vi "Ballard 429 - Parse Message.vi"(8 "Error (in)":errorcluster, 9 "Data (in)":dbl[](array[numeric]), 10 "Record []":T13[](array[typedef]) {"type" format="%04x"; "timestamp" format="%08x"; "msgact" format="%04x"; "data" format="%08x"; "timestamph" format="%08x"}, 11 "Channel Data []":T1[](array[typedef])=[{"Labels Settings"=[{"Name"="", "xmlName"="", "Label"=0, "transferPeriod"=0, "Driver Data"={"Lbl Tx Hdl"=0, "Decimation"=0, "IterationOffset"=0, "transfer handle"=0, "RX Word"=0, "TXChange"=FALSE, "RX timestamp"=0.0}, "SDI_Enabled"=FALSE, "SDI"=0, "Words"=[{"Block Data Refs"=[], "Values Array"=[], "Length"=0, "FIFO Index"=0, "Param Setting"={"Start Bit"=[1], "Num Bits"=[], "Signed?"=[], "ScaleFac"=[], "ScaleOffset"=[], "Channel FIFO Buffer Index"=[]}}], "bufferSize"=0, "RxWordIdx"=0, "TxWordIdx"=0, "TransferType"=enum."ScheduledLabel", "has timestamp?"=FALSE, "LBL Disable Index"=0, "Message Handle"=0, "Initialized?"=FALSE}], "channel handle"=0, "channel #"=0, "Label Map"=[], "Label Buffer"=[], "rdBufHandle"=0}] {"Labels Settings"."Label" format="%.0o"}) -> (0 "Error (out)":errorcluster, 1 "Doubles []":dbl[](array[numeric]))   [LabVIEW 2017, in "Ballard Arinc-429 Engine.lvlib"]
uses:
  Ballard Arinc-429 Engine.lvlib
  <instrlib>/BTICardLib/Public/Controls/429 Record.ctl
  RT Controls/RT HW Channel.ctl
  RT Controls/RT Label Settings.ctl
  Shared/Controls and Global/Label.ctl
  Shared/Controls and Global/transferPeriod.ctl
  RT Controls/Driver Data.ctl
  RT Controls/RT Word Settings.ctl
  <vilib>/NI Veristand/Custom Device API/Block Data Reference.ctl
  <vilib>/NI Veristand/Custom Device API/Data Reference.ctl
  RT Controls/RT Param Setting.ctl
  Shared/Controls and Global/Start Bit.ctl
  Shared/Controls and Global/Number of Bits.ctl
  Shared/Controls and Global/TransferType.ctl
  <instrlib>/BTI429Lib/BTI429LV.lvlib
  Shared/Ballard Arinc-429 Shared.lvlib
  <instrlib>/BTI429Lib/Private/Utility/Get Fld SDI.vi
  <instrlib>/BTICardLib/BTICardLV.lvlib
  <vilib>/NI Veristand/Custom Device API/Custom Device API.lvlib
panel:
  out "Waveform Chart":i32(graph)
  out "source/destination identifiers (SDI) out":u8 format="%02b"
  out "Label #":i32
  out "Physical Channel #":i32
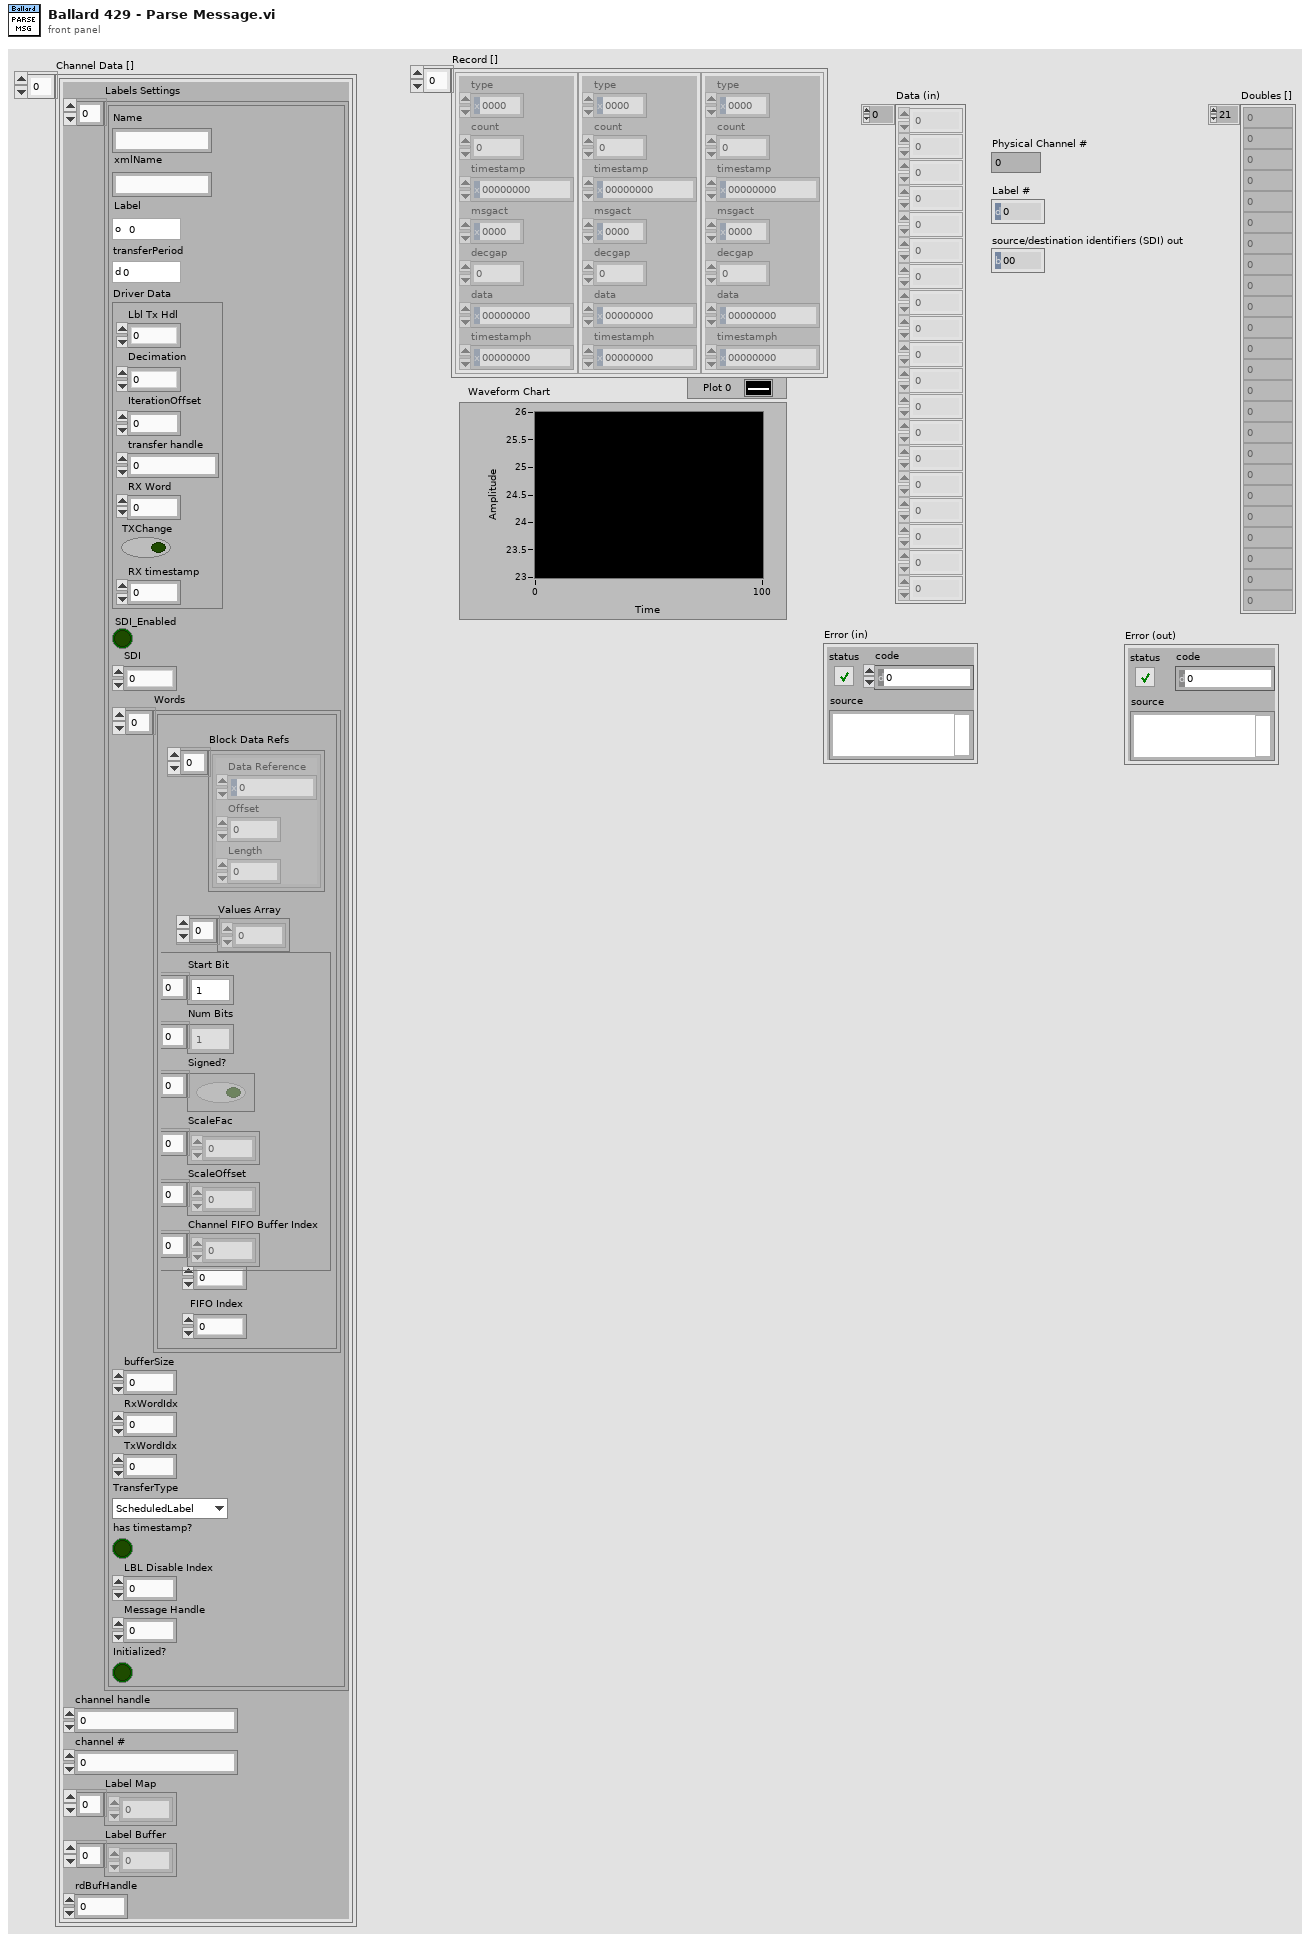
[diagram p1: front panel]
types:
  T1 = typedef "Ballard Arinc-429 Engine.lvlib/RT HW Channel.ctl" = cluster{"Labels Settings":T2[], "channel handle":u32, "channel #":u16, "Label Map":i32[], "Label Buffer":u32[], "rdBufHandle":u32}
  T2 = typedef "Ballard Arinc-429 Engine.lvlib/RT Label Settings.ctl" = cluster{"Name":string, "xmlName":string, "Label":T3, "transferPeriod":T4, "Driver Data":T5, "SDI_Enabled":bool, "SDI":u8, "Words":T6[], "bufferSize":u32, "RxWordIdx":i32, "TxWordIdx":i32, "TransferType":T12, "has timestamp?":bool, "LBL Disable Index":i32, "Message Handle":u64, "Initialized?":bool}
  T3 = typedef "Ballard Arinc-429 Shared.lvlib/Label.ctl" = u8
  T4 = typedef "Ballard Arinc-429 Shared.lvlib/transferPeriod.ctl" = u32
  T5 = typedef "Ballard Arinc-429 Engine.lvlib/Driver Data.ctl" = cluster{"Lbl Tx Hdl":u32, "Decimation":i32, "IterationOffset":i32, "transfer handle":u32, "RX Word":u32, "TXChange":bool, "RX timestamp":dbl}
  T6 = typedef "Ballard Arinc-429 Engine.lvlib/RT Word Settings.ctl" = cluster{"Block Data Refs":T7[], "Values Array":dbl[], "Length":i32, "FIFO Index":i32, "Param Setting":T9}
  T7 = typedef "Custom Device API.lvlib/Block Data Reference.ctl" = cluster{"Data Reference":T8, "Offset":u64, "Length":u64}
  T8 = typedef "Custom Device API.lvlib/Data Reference.ctl" = i32
  T9 = typedef "Ballard Arinc-429 Engine.lvlib/RT Param Setting.ctl" = cluster{"Start Bit":T10[], "Num Bits":T11[], "Signed?":bool[], "ScaleFac":dbl[], "ScaleOffset":dbl[], "Channel FIFO Buffer Index":i32[]}
  T10 = typedef "Ballard Arinc-429 Shared.lvlib/Start Bit.ctl" = i32
  T11 = typedef "Ballard Arinc-429 Shared.lvlib/Number of Bits.ctl" = i32
  T12 = typedef "Ballard Arinc-429 Shared.lvlib/TransferType.ctl" = enum16{"ScheduledLabel", "Acyclic", "Block", "Strobe"}
  T13 = typedef "BTICardLV.lvlib/429 Record.ctl" = cluster{"type":u16, "count":u16, "timestamp":u32, "msgact":u16, "decgap":u16, "data":u32, "timestamph":u32}
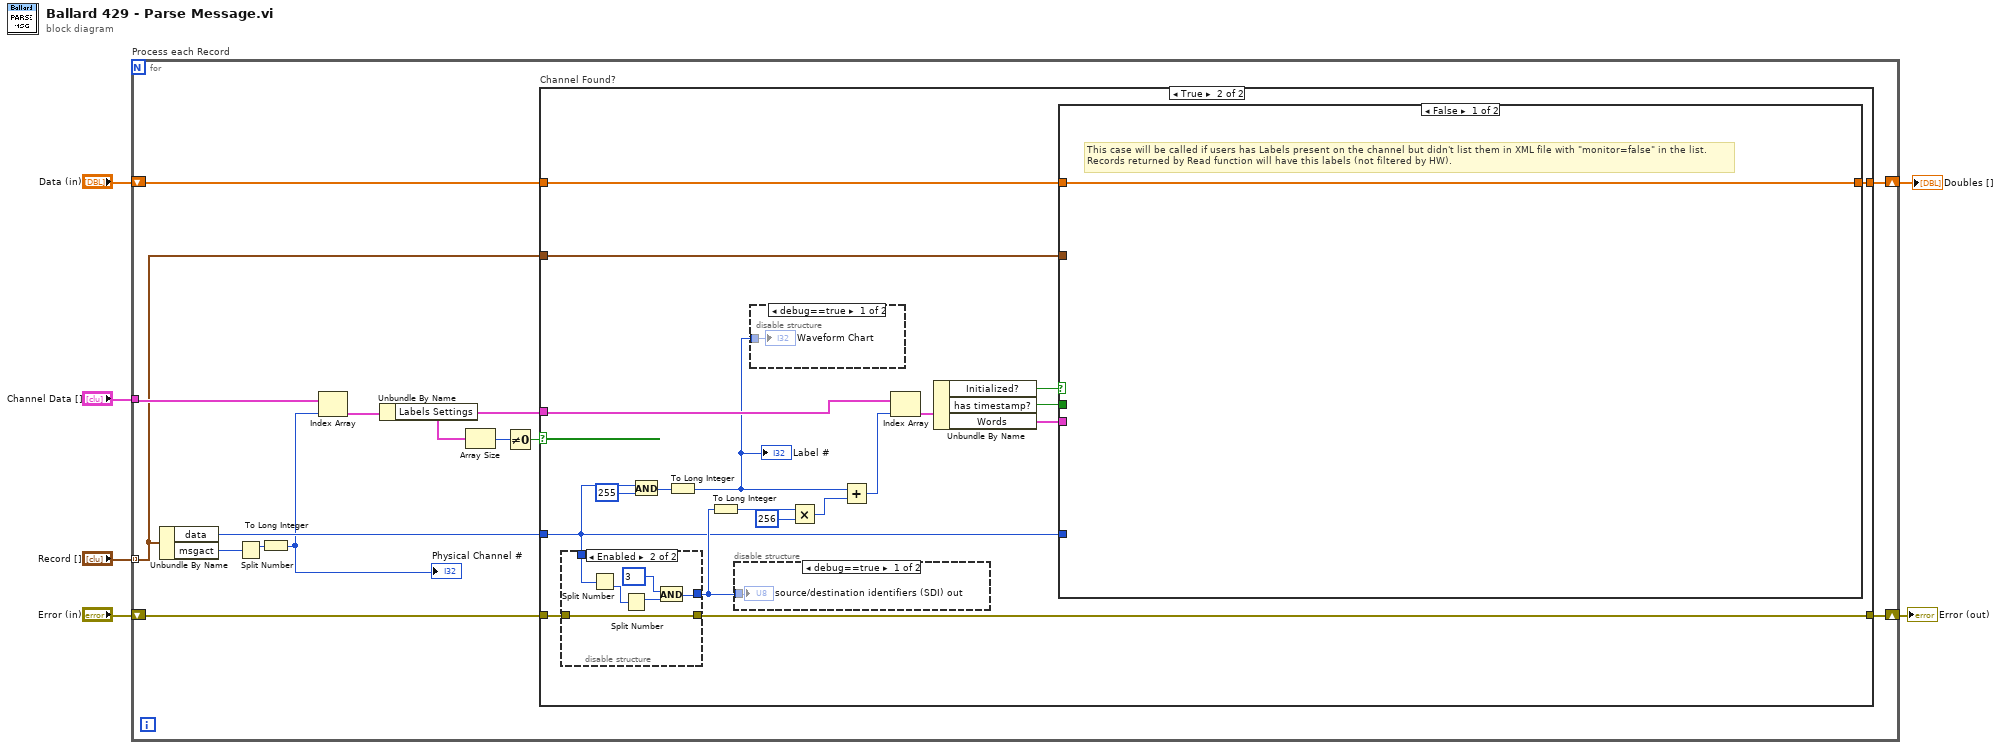
[diagram p0: block diagram]
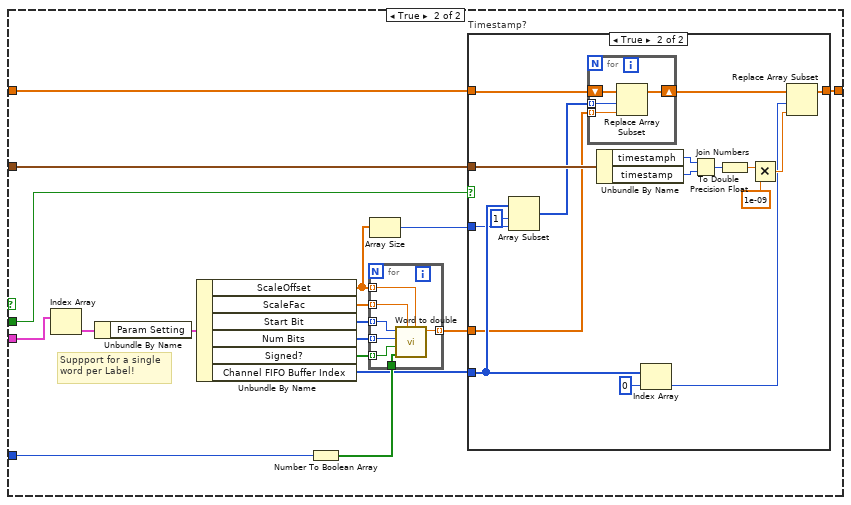
[diagram p3: hidden frame]
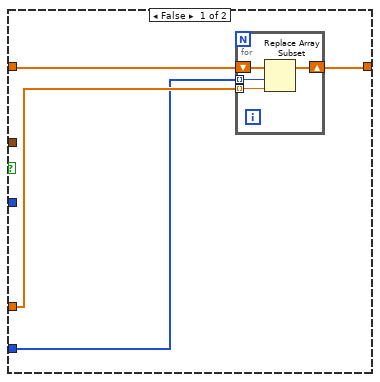
[diagram p4: hidden frame]
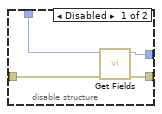
[diagram p7: hidden frame]
diagram:
  n1 = for "Process each Record" {
    tunnel: "Record []" -> [w14] mode=indexing
    shift-right: [w19] -> w3
    shift-left: "Error (in)" -> [w20]
    tunnel: "Channel Data []" -> [w16]
    shift-right: [w7] -> w1
    shift-left: "Data (in)" -> [w11]
    n2 = Unbundle By Name(w14) -> ("data"=w17:u32, "msgact"=w13:u16)
    n3 = Split Number(x=w13) -> (hi(x)=w9:u8)  [unwired: 1 out]
    n4 = To Long Integer(number=w9) -> (32bit integer=w12:i32)
    "Physical Channel #" <- w12
    n5 = Index Array(array=w16, index=w12) -> (element=w15:T1)
    n6 = Unbundle By Name(w15) -> ("Labels Settings"=w8:T2[])
    n7 = Array Size(array=w8) -> (size(s)=w10:i32)
    n8 = Not Equal To 0?(x=w10) -> (x != 0?=w18:bool)
    n9 = case "Channel Found?" shown="True" w18 {
      tunnel: w20 -> [w22 w36]
      tunnel: [w22 w41] -> w19
      tunnel: w17 -> [_ w25]
      tunnel: w14 -> [_ w39]
      tunnel: w11 -> [w21 w27]
      tunnel: w8 -> [_ w33]
      tunnel: [w21 w26] -> w7
      frame False {
      }
      frame True {
        n10 = disable-structure shown="Enabled" {
          disable-tunnel: w25 -> [w101 w106]
          disable-tunnel: w36 -> [w100 w107]
          disable-tunnel: [w99 w107] -> w41
          disable-tunnel: [w98 w104] -> w35
          frame Disabled {
            n11 = call-poly <instrlib>:"Get Fields.vi"("error in (no error)"=w100, "message"=w101) -> ("error out"=w99:errorcluster, "source/destination identifiers (SDI) out"=w98:u16)  [unwired: 8 in]
          }
          frame Enabled {
            n12 = Split Number(x=w106) -> (lo(x)=w105:u16)  [unwired: 1 out]
            n13 = Split Number(x=w105) -> (hi(x)=w103:u8)  [unwired: 1 out]
            n14 = And(x=u8 3, y=w103) -> (x .and. y?=w104:u8)
          }
        }
        n15 = And(x=w25, y=u32 255) -> (x .and. y?=w37:u32)
        n16 = To Long Integer(number=w37) -> (32bit integer=w24:i32)
        "Label #" <- w24
        n17 = To Long Integer(number=w35) -> (32bit integer=w34:i32)
        n18 = disable-structure shown="debug==true" {
          disable-tunnel: w35 -> [w96 _]
          frame condition #0 {
            "source/destination identifiers (SDI) out" <- w96
          }
          frame condition #1 (active) {
          }
        }
        n19 = disable-structure shown="debug==true" {
          disable-tunnel: w24 -> [w97 _]
          frame condition #0 {
            "Waveform Chart" <- w97
          }
          frame condition #1 (active) {
          }
        }
        n20 = Multiply(x=w34, y=256) -> (x*y=w32:i32)
        n21 = Add(x=w24, y=w32) -> (x+y=w31:i32)
        n22 = Index Array(array=w33, index=w31) -> (element=w29:T2)
        n23 = Unbundle By Name(w29) -> ("Initialized?"=w23:bool, "has timestamp?"=w38:bool, "Words"=w40:T6[])
        n24 = case shown="False" w23 {
          tunnel: w40 -> [_ w59]
          tunnel: w39 -> [_ w58]
          tunnel: w38 -> [_ w57]
          tunnel: w27 -> [w42 w49]
          tunnel: [w42 w48] -> w26
          tunnel: w25 -> [_ w47]
          frame False {
            # "This case will be called if users has Labels present on the channel but didn't list them in XML file with \"monitor=false\" in the list.\nRecords returned by Read function will have this labels (not filtered by HW)."
          }
          frame True {
            # "Suppport for a single\nword per Label!"
            n25 = Index Array(array=w59) -> (element=w56:T6)  [unwired: 1 in]
            n26 = Unbundle By Name(w56) -> ("Param Setting"=w55:T9)
            n27 = Unbundle By Name(w55) -> ("ScaleOffset"=w44:dbl[], "ScaleFac"=w54:dbl[], "Start Bit"=w53:T10[], "Num Bits"=w52:T11[], "Signed?"=w51:bool[], "Channel FIFO Buffer Index"=w45:i32[])
            n28 = Number To Boolean Array(number=w47) -> (Boolean array=w46:bool[])
            n29 = for {
              tunnel: [w95] -> w50 mode=indexing
              tunnel: w44 -> [w94] mode=indexing
              tunnel: w54 -> [w93] mode=indexing
              tunnel: w53 -> [w92] mode=indexing
              tunnel: w52 -> [w91] mode=indexing
              tunnel: w51 -> [w90] mode=indexing
              tunnel: w46 -> [w89]
              n30 = call "Word to double.vi"("ScaleOffset (0)"=w94, "ScaleFac (1)"=w93, "Word"=w89, "Signed? (F)"=w90, "Number of Bits"=w91, "Start Bit"=w92) -> ("Double"=w95:dbl)  [unwired: 5 in]
            }
            n31 = Array Size(array=w44) -> (size(s)=w43:i32)
            n32 = case "Timestamp?" shown="True" w57 {
              tunnel: w50 -> [w61 w68]
              tunnel: w58 -> [_ w79]
              tunnel: w49 -> [w63 w76]
              tunnel: [w62 w78] -> w48
              tunnel: w45 -> [w60 w72]
              tunnel: w43 -> [_ w70]
              frame False {
                n33 = for {
                  shift-right: [w66] -> w62
                  shift-left: w63 -> [w67]
                  tunnel: w61 -> [w65] mode=indexing
                  tunnel: w60 -> [w64] mode=indexing
                  n34 = Replace Array Subset(array=w67, new element=w65, index=w64) -> (w66:dbl[])
                }
              }
              frame True {
                n35 = Array Subset(array=w72, index=1, length=w70) -> (w69:i32[])
                n36 = for {
                  shift-right: [w87] -> w75
                  shift-left: w76 -> [w88]
                  tunnel: w68 -> [w86] mode=indexing
                  tunnel: w69 -> [w85] mode=indexing
                  n37 = Replace Array Subset(array=w88, new element=w86, index=w85) -> (w87:dbl[])
                }
                n38 = Unbundle By Name(w79) -> ("timestamph"=w84:u32, "timestamp"=w83:u32)
                n39 = Index Array(array=w72, index=0) -> (element=w73:i32)
                n40 = Join Numbers(hi=w84, lo=w83) -> ((hi.lo)=w82:u64)
                n41 = To Double Precision Float(number=w82) -> (double precision float=w81:dbl)
                n42 = Multiply(x=w81, y=1e-09) -> (x*y=w77:dbl)
                n43 = Replace Array Subset(array=w75, new element=w77, index=w73) -> (w78:dbl[])
              }
            }
          }
        }
      }
    }
  }
  "Error (out)" <- w3
  "Doubles []" <- w1
